vi "Gyro Globals.vi"() -> ()   [LabVIEW 2014]
panel:
  in  "Reset?":bool
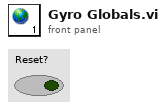
[diagram p1: front panel]
diagram:
